vi "波形描述检查.vi"(11 "波形描述":string[][](array[string])) -> (2 "不正确?":bool, 3 "波形描述输出":string[][](array[string]))   [LabVIEW 2020, in "功能选择.xctl"]
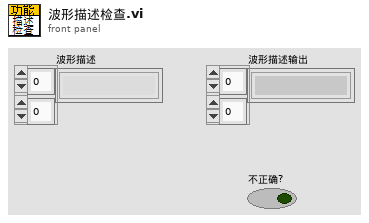
[diagram p1: front panel]
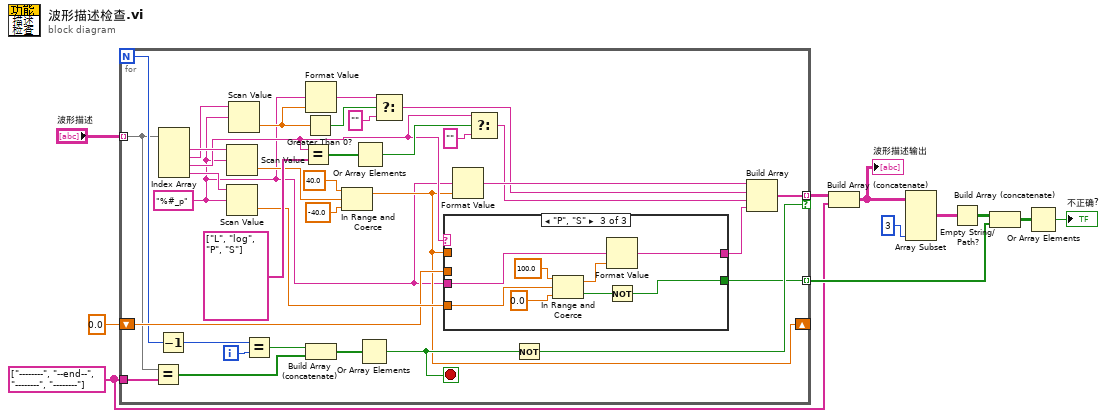
[diagram p0: block diagram]
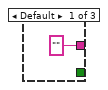
[diagram p2: hidden frame]
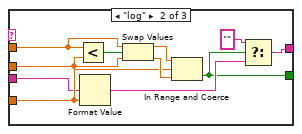
[diagram p3: hidden frame]
diagram:
  w3 = string[] ["--------", "--end--", "--------", "--------"] ("波形描述")
  n1 = for {
    N -> [w22]
    tunnel: "波形描述" -> [w15] mode=indexing
    shift-right: [w17] -> _
    shift-left: 0.0 -> [w27]
    tunnel: [w26] -> w2 mode=indexing if=w23
    tunnel: w3 -> [w14]
    tunnel: [w13] -> w9 mode=indexing
    i -> [w21]
    stop <- w24 stop-if-true
    w12 = "%#_p" ("格式字符串")
    n2 = Equal?(x=w15, y=w14) -> (x = y?=w25:bool[])
    n3 = Decrement(x=w22) -> (x-1=w20:i32)
    n4 = Index Array(array=w15) -> (element #1=w46:string, element #2=w45:string, element #3=w30:string, element #4=w44:string)  [unwired: 4 in]
    n5 = Scan Value(string=w46, format string=w12) -> (value=w28:dbl)  [unwired: 1 in, 1 out]
    n6 = Scan Value(string=w44, format string=w12) -> (value=w31:dbl)  [unwired: 1 in, 1 out]
    n7 = Scan Value(string=w45, format string=w12) -> (value=w16:dbl)  [unwired: 1 in, 1 out]
    n8 = Equal?(x=w20, y=w21) -> (x = y?=w18:bool)
    n9 = Equal?(x=w30, y=string[] ["L", "log", "P", "S"] ("NewVal")) -> (x = y?=w40:bool[])
    n10 = Greater Than 0?(x=w16) -> (x > 0?=w35:bool)
    n11 = Format Value(format string=w12, value (0)=w16) -> (output string=w34:string)  [unwired: 1 in]
    n12 = Build Array (concatenate)(w18, w25) -> (w19:bool[])
    n13 = In Range and Coerce(upper limit=40.0 ("上限"), x=w28, lower limit=-40.0 ("下限")) -> (coerced(x)=w17:dbl)  [unwired: 1 out]
    n14 = Or Array Elements(Boolean array=w40) -> (logical OR=w39:bool)
    n15 = Or Array Elements(Boolean array=w19) -> (logical OR=w24:bool)
    n16 = Select(t=w34, s=w35, f="") -> (s? t:f=w32:string)
    n17 = case shown="\"P\", \"S\"" w30 {
      tunnel: w31 -> [_ w50 w64]
      tunnel: ["" w51 w63] -> w29
      tunnel: w17 -> [_ w58 _]
      tunnel: w27 -> [_ w57 _]
      tunnel: w12 -> [_ w49 w61]
      tunnel: [_ w48 w59] -> w13
      frame Default {
      }
      frame "log" {
        n18 = Less?(x=w58, y=w57) -> (x < y?=w56:bool)
        n19 = Format Value(format string=w49, value (0)=w50) -> (output string=w52:string)  [unwired: 1 in]
        n20 = Swap Values(12:w58, 13:w56, 14:w57) -> (1:w54:dbl, 3:w55:dbl)
        n21 = In Range and Coerce(upper limit=w54, x=w50, lower limit=w55) -> (In Range?=w48:bool)  [unwired: 1 out]
        n22 = Select(t="", s=w48, f=w52) -> (s? t:f=w51:string)
      }
      frame "P", "S" {
        n23 = In Range and Coerce(upper limit=100.0 ("上限"), x=w64, lower limit=0.0 ("下限")) -> (coerced(x)=w62:dbl, In Range?=w60:bool)
        n24 = Format Value(format string=w61, value (0)=w62) -> (output string=w63:string)  [unwired: 1 in]
        n25 = Not(x=w60) -> (.not. x?=w59:bool)
      }
    }
    n26 = Format Value(format string=w12, value (0)=w17) -> (output string=w41:string)  [unwired: 1 in]
    n27 = Select(t=w30, s=w39, f="") -> (s? t:f=w36:string)
    n28 = Not(x=w24) -> (.not. x?=w23:bool)
    n29 = Build Array(w41, w32, w36, w29) -> (w26:string[])
  }
  n30 = Build Array (concatenate)(w2, w3) -> (w11:string[][])
  "波形描述输出" <- w11
  n31 = Array Subset(array=w11, length (col)=3 ("长度")) -> (w5:string[][])  [unwired: 3 in]
  n32 = Empty String/Path?(string/path=w5) -> (empty?=w6:bool[][])
  n33 = Build Array (concatenate)(w6, w9) -> (w8:bool[][])
  n34 = Or Array Elements(Boolean array=w8) -> (logical OR=→"不正确?":bool)
